vi "PhotonPNPResult_unpackt.vi"(9 "StartByte":i32, 11 "RawData":u8[](array[numeric])) -> (1 "NextByte":i32, 3 "PNP_Result":T1={"IsPresent"=FALSE, "bestReprojErr"=0.0, "altReprojErr"=0.0, "ambiguity"=0.0, "Best"={"TRANSLATION3D"={"X"=0.0, "Y"=0.0, "Z"=0.0}, "ROTATION3D"={"Q_quaternion"={"R"=1.0, "V"=[0.0, 0.0, 0.0]}}, "XF"=FALSE}, "Alt"={"TRANSLATION3D"={"X"=0.0, "Y"=0.0, "Z"=0.0}, "ROTATION3D"={"Q_quaternion"={"R"=1.0, "V"=[0.0, 0.0, 0.0]}}, "XF"=FALSE}} {"Alt"."TRANSLATION3D"."Z" format="%14.3f"; "Alt"."TRANSLATION3D"."Y" format="%14.3f"; "Alt"."TRANSLATION3D"."X" format="%14.3f"; "Best"."TRANSLATION3D"."Z" format="%14.3f"; "Best"."TRANSLATION3D"."Y" format="%14.3f"; "Best"."TRANSLATION3D"."X" format="%14.3f"})   [LabVIEW 2019, in "PhotonVisionLib.lvlib"]
doc: "Internal function to parse the data for each target returned by PhotonCamera_GetLatestResult.\n\nInputs:\n - RawData -- Byte array containing the data to parse.\n\nOutputs:\n - TrackedTarget -- Parsed TrackedTarget cluster."
uses:
  <vilib>/Rock Robotics/WPI/ThirdParty/JAS_Junk/TrajLib/VI/Transform3d_Create_Trans3dRot3d.vi
  <vilib>/Rock Robotics/WPI/ThirdParty/JAS_Junk/TrajLib/VI/Translation3d_Create.vi
  <vilib>/Rock Robotics/WPI/ThirdParty/JAS_Junk/TrajLib/VI/Rotation3d_Create_Quaternion.vi
  <vilib>/Rock Robotics/WPI/ThirdParty/JAS_Junk/TrajLib/VI/Quaternion_New.vi
  <vilib>/Rock Robotics/WPI/ThirdParty/JAS_Junk/TrajLib/VI/Quaternion_Normalize.vi
  <vilib>/Rock Robotics/WPI/ThirdParty/JAS_Junk/TrajLib/VI/Quaternion_New_Default.vi
  PhotonVisionLib.lvlib
  <vilib>/Rock Robotics/WPI/ThirdParty/JAS_Junk/TrajLib/TypeDef/TRANSLATION3D.ctl
  <vilib>/Rock Robotics/WPI/ThirdParty/JAS_Junk/TrajLib/Trajectory_Library.lvlib
  <vilib>/Rock Robotics/WPI/ThirdParty/JAS_Junk/TrajLib/TypeDef/QUATERNION.ctl
  <vilib>/Rock Robotics/WPI/ThirdParty/JAS_Junk/TrajLib/TypeDef/ROTATION3D.ctl
  <vilib>/Rock Robotics/WPI/ThirdParty/JAS_Junk/TrajLib/TypeDef/TRANSFORM3D.ctl
  TypeDef/PhotonPNPResult.ctl
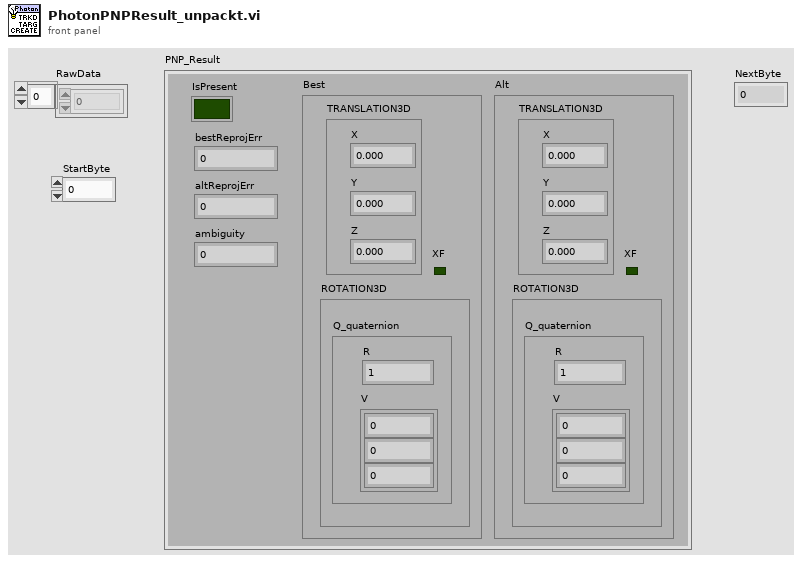
[diagram p1: front panel]
types:
  T1 = typedef "PhotonVisionLib.lvlib/PhotonPNPResult.ctl" = cluster{"IsPresent":bool, "bestReprojErr":dbl, "altReprojErr":dbl, "ambiguity":dbl, "Best":T2, "Alt":T2}
  T2 = typedef "Trajectory_Library.lvlib/TRANSFORM3D.ctl" = cluster{"TRANSLATION3D":T3, "ROTATION3D":T4, "XF":bool}
  T3 = typedef "Trajectory_Library.lvlib/TRANSLATION3D.ctl" = cluster{"X":dbl, "Y":dbl, "Z":dbl}
  T4 = typedef "Trajectory_Library.lvlib/ROTATION3D.ctl" = cluster{"Q_quaternion":T5}
  T5 = typedef "Trajectory_Library.lvlib/QUATERNION.ctl" = cluster{"R":dbl, "V":dbl[]}
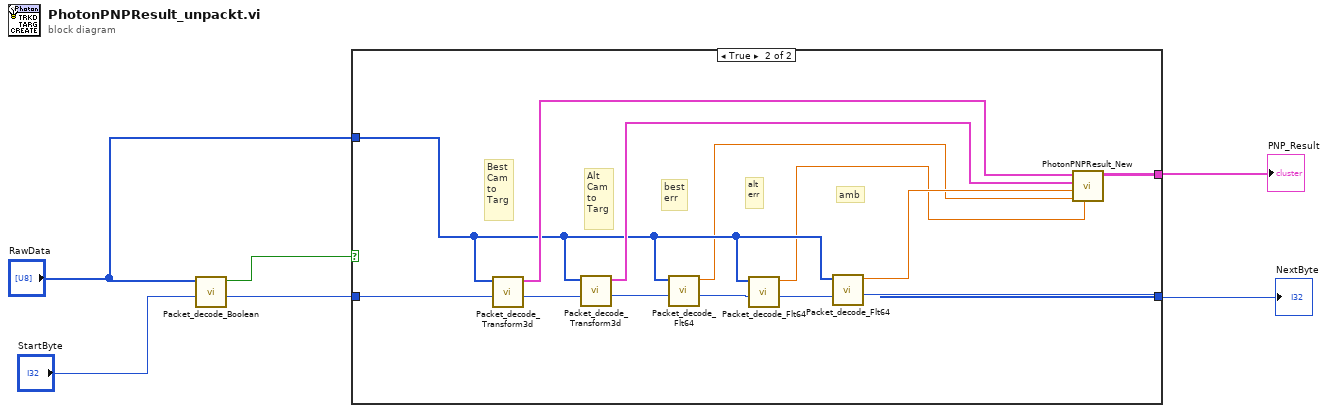
[diagram p0: block diagram]
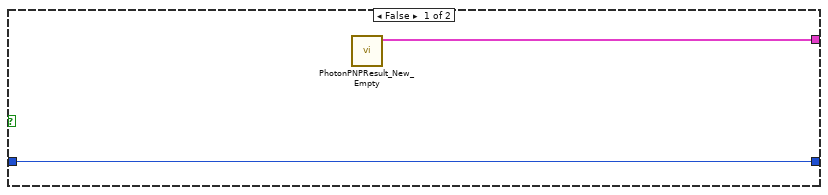
[diagram p2: hidden frame]
diagram:
  n1 = call "Packet_decode_Boolean.vi"("StartByte"="StartByte", "RawData"="RawData") -> ("NextByte"=w4:i32, "Boolean_Value"=w5:bool)  [unwired: 8 in]
  n2 = case shown="True" w5 {
    tunnel: w4 -> [w8 w19]
    tunnel: [w8 w14] -> w3
    tunnel: [w7 w9] -> w2
    tunnel: "RawData" -> [_ w13]
    frame False {
      n3 = call "PhotonPNPResult_New_Empty.vi"() -> ("PNP_Result"=w7:T1)  [unwired: 11 in]
    }
    frame True {
      # "amb"
      # "alt\nerr"
      # "best\nerr"
      # "Alt\nCam\nto\nTarg"
      # "Best\nCam\nto\nTarg"
      n4 = call "Packet_decode_Transform3d.vi"("NextByte in"=w19, "RawData"=w13) -> ("NextByte out"=w20:i32, "Transform3d"=w18:T2)  [unwired: 6 in]
      n5 = call "Packet_decode_Transform3d.vi"("NextByte in"=w20, "RawData"=w13) -> ("NextByte out"=w21:i32, "Transform3d"=w17:T2)  [unwired: 6 in]
      n6 = call "Packet_decode_Flt64.vi"("StartByte"=w21, "RawData"=w13) -> ("NextByte"=w16:i32, "Flt64_Value"=w11:dbl)  [unwired: 8 in]
      n7 = call "Packet_decode_Flt64.vi"("StartByte"=w16, "RawData"=w13) -> ("NextByte"=w15:i32, "Flt64_Value"=w10:dbl)  [unwired: 8 in]
      n8 = call "Packet_decode_Flt64.vi"("StartByte"=w15, "RawData"=w13) -> ("NextByte"=w14:i32, "Flt64_Value"=w12:dbl)  [unwired: 8 in]
      n9 = call "PhotonPNPResult_New.vi"("altReprojErr"=w10, "bestReprojErr"=w11, "ambiguity"=w12, "Alt"=w17, "Best"=w18) -> ("PNP_Result"=w9:T1)  [unwired: 6 in]
    }
  }
  "PNP_Result" <- w2
  "NextByte" <- w3
